vi "Wait on Abort.vi"(8 "error in (no error)":errorcluster, 9 "timeout in ms (0)":i32, 11 "Slave Test Runner In":refnum<class "Slave Test Runner.lvclass">) -> (0 "error out":errorcluster, 1 "Aborted?":bool, 3 "Slave Test Runner Out":refnum<class "Slave Test Runner.lvclass">)   [LabVIEW 2020, in "Slave Test Runner.lvclass"]
doc: "Check the abort notifier."
uses:
  Slave Test Runner.lvclass
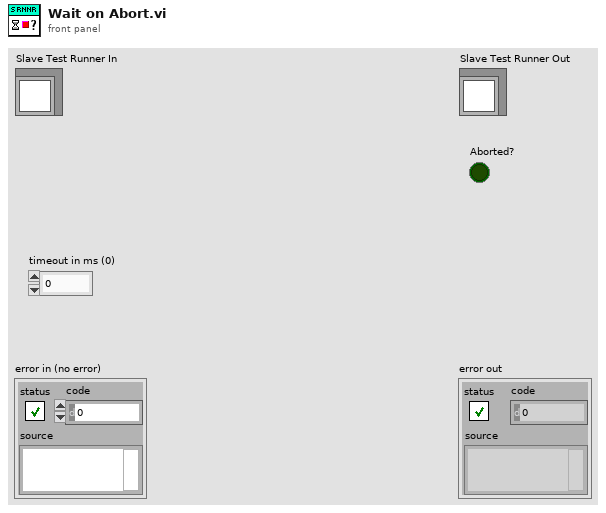
[diagram p1: front panel]
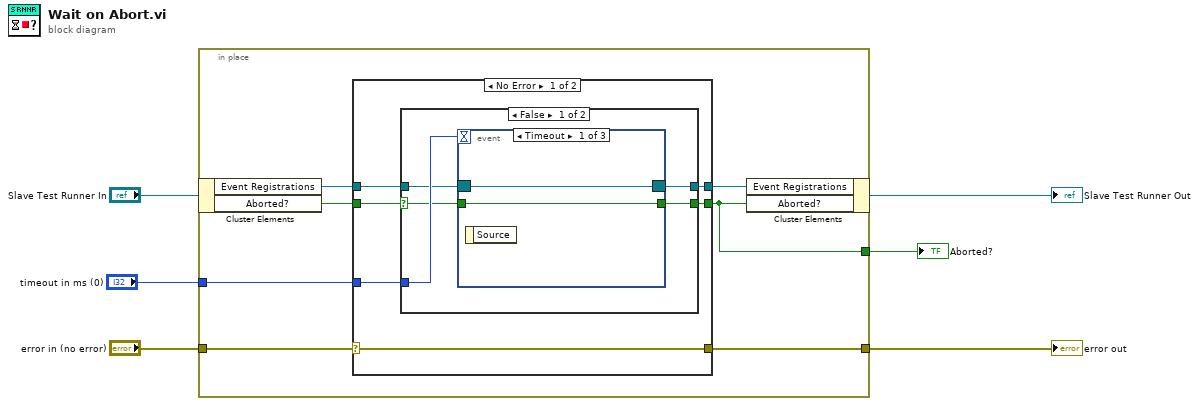
[diagram p0: block diagram]
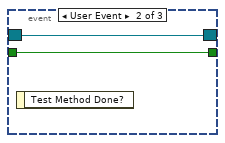
[diagram p2: hidden frame]
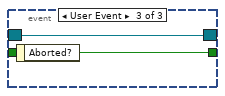
[diagram p3: hidden frame]
diagram:
  n1 = in-place {
    in-place-border: "error in (no error)" -> [w13]
    in-place-border: "timeout in ms (0)" -> [w12]
    in-place-border: [w7] -> w2
    in-place-border: [w8] -> w1
    n2 = in-place-cluster #1("Slave Test Runner In") -> ("Event Registrations"=w11:refnum<event-registration>, "Aborted?"=w10:bool)
    n3 = case shown="No Error" w13 {
      selector: w13 -> [w14 w33]
      tunnel: w10 -> [w19 w34]
      tunnel: w12 -> [w18 _]
      tunnel: w11 -> [w17 w35]
      tunnel: [w16 w35] -> w9
      tunnel: [w15 w34] -> w7
      tunnel: [w14 w33] -> w8
      frame No Error {
        n4 = case shown="False" w19 {
          selector: w19 -> [w20 w31]
          tunnel: w18 -> [w24 _]
          tunnel: w17 -> [w23 w32]
          tunnel: [w22 w32] -> w16
          tunnel: [w21 w31] -> w15
          frame False {
            n5 = event shown="[0] Timeout" {
              selector: w23 -> [w26 w27 w29]
              dyn-events: [w26 w27 w29] -> w22
              timeout: w24 -> [_ _ _]
              tunnel: [w25 w28 w30] -> w21
              tunnel: w20 -> [w25 w28 _]
              event Timeout {
                n6 = event-data() -> ()  [unwired: 1 in, 1 out]
              }
              event User Event {
                n7 = event-data() -> ()  [unwired: 1 in, 1 out]
              }
              event User Event {
                n8 = event-data() -> ("Aborted?"=w30:bool)  [unwired: 1 in]
              }
            }
          }
          frame True {
          }
        }
      }
      frame Error {
      }
    }
    n9 = in-place-cluster #1("Event Registrations"=w9, "Aborted?"=w7) -> (→"Slave Test Runner Out":refnum<class "Slave Test Runner.lvclass">)
  }
  "error out" <- w1
  "Aborted?" <- w2
